vi "ANAL_BinSummer.vi"(6 "Sweep Range":cluster{"Numeric":i32, "Numeric":i32}, 8 "No. Cycles":u32, 9 "Target Set Points":i32[](array[numeric]), 10 "Software Gate":cluster{"Numeric":i32, "Numeric":i32}, 11 "Run Data Cluster":T1 {"Temperature B" scale=0.0..100.0; "Temperature A" scale=0.0..100.0}) -> (1 "Sweeps":i32, 2 "PackedArray":i32[][](array[numeric]))   [LabVIEW 2021]
uses:
  DAT_Cluster.ctl
  81de8623-b3e4-400a-9ecc-59d5fbcc5fd3.vi
  81de8623-b3e4-400a-9ecc-59d5fbcc5fd3.vi/d4db2432-cc9c-482c-8957-dac855435ef6.vi
  81de8623-b3e4-400a-9ecc-59d5fbcc5fd3.vi/86fbf154-bd7b-49a2-8ab2-a837b2a95f24.vi
  81de8623-b3e4-400a-9ecc-59d5fbcc5fd3.vi/3b95b01e-1ec2-4565-bcd9-7606a5281010.vi
  81de8623-b3e4-400a-9ecc-59d5fbcc5fd3.vi/96a08935-737a-44b2-979c-a81d56408f7e.vi
  81de8623-b3e4-400a-9ecc-59d5fbcc5fd3.vi/d4db2432-cc9c-482c-8957-dac855435ef6.vi/6eaecd13-6e48-4772-a921-b51ebdf84d88.vi
  81de8623-b3e4-400a-9ecc-59d5fbcc5fd3.vi/d4db2432-cc9c-482c-8957-dac855435ef6.vi/d2d5f2b7-06f4-47f6-971c-049c3fdbb653.vi
  81de8623-b3e4-400a-9ecc-59d5fbcc5fd3.vi/3b95b01e-1ec2-4565-bcd9-7606a5281010.vi/6eaecd13-6e48-4772-a921-b51ebdf84d88.vi
  81de8623-b3e4-400a-9ecc-59d5fbcc5fd3.vi/3b95b01e-1ec2-4565-bcd9-7606a5281010.vi/d2d5f2b7-06f4-47f6-971c-049c3fdbb653.vi
  81de8623-b3e4-400a-9ecc-59d5fbcc5fd3.vi/96a08935-737a-44b2-979c-a81d56408f7e.vi/6eaecd13-6e48-4772-a921-b51ebdf84d88.vi
  81de8623-b3e4-400a-9ecc-59d5fbcc5fd3.vi/96a08935-737a-44b2-979c-a81d56408f7e.vi/d2d5f2b7-06f4-47f6-971c-049c3fdbb653.vi
  <vilib>/Comparison/Less/Less Functor/Less Functor.lvclass
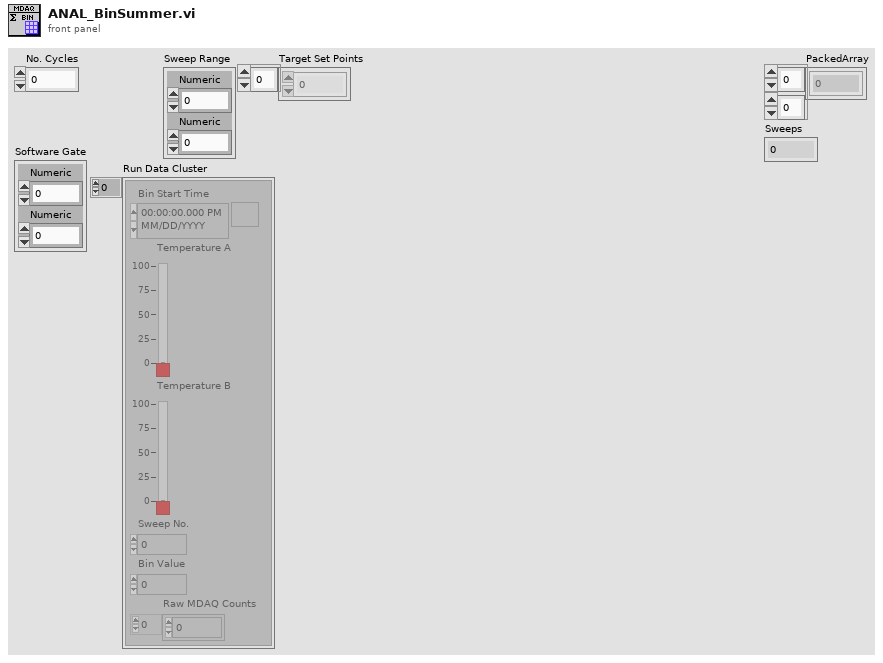
[diagram p1: front panel]
types:
  T1 = typedef "DAT_Cluster.ctl" = cluster{"Bin Start Time":timestamp, "Temperature A":dbl, "Temperature B":dbl, "Sweep No.":i32, "Bin Value":i32, "Raw MDAQ Counts":i32[]}[]
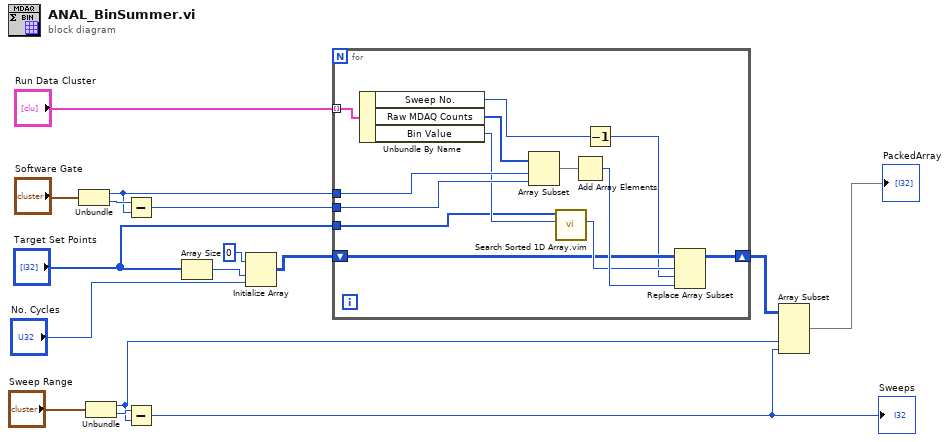
[diagram p0: block diagram]
diagram:
  n1 = Unbundle("Software Gate") -> ("Numeric"=w13:i32, "Numeric"=w14:i32)
  n2 = Unbundle("Sweep Range") -> ("Numeric"=w3:i32, "Numeric"=w4:i32)
  n3 = Subtract(x=w14, y=w13) -> (x-y=w12:i32)
  n4 = Subtract(x=w4, y=w3) -> (x-y=w2:i32)
  "Sweeps" <- w2
  n5 = Array Size(array="Target Set Points") -> (size(s)=w10:i32)
  n6 = Initialize Array(0 ("element"), w10, "No. Cycles") -> (w9:i32[][])
  n7 = for {
    tunnel: "Run Data Cluster" -> [w29] mode=indexing
    tunnel: w13 -> [w27]
    tunnel: w12 -> [w26]
    shift-right: [w20] -> w6
    shift-left: w9 -> [w21]
    tunnel: "Target Set Points" -> [w17]
    n8 = Unbundle By Name(w29) -> ("Sweep No."=w19:i32, "Raw MDAQ Counts"=w28:i32[], "Bin Value"=w23:i32)
    n9 = Array Subset(array=w28, index=w27, length=w26) -> (w25:i32[])
    n10 = call "Search Sorted 1D Array.vim"("element"=w23, "sorted 1D array"=w17) -> ("nearest index"=w22:i32)  [unwired: 8 in, 1 out]
    n11 = Add Array Elements(numeric array=w25) -> (sum=w24:i32)
    n12 = Decrement(x=w19) -> (x-1=w18:i32)
    n13 = Replace Array Subset(array=w21, new element=w24, index (row)=w22, index (col)=w18) -> (w20:i32[][])
  }
  n14 = Array Subset(array=w6, index (col)=w3, length (col)=w2) -> (→"PackedArray":i32[][])  [unwired: 2 in]
